vi "Lift Joystick Get.vi"(8 "Button Index's":T2, 9 "Setpoints":T1, 10 "Joystick IN":bool[](array[boolean]), 11 "Position IN":dbl format="%#_13g") -> (2 "Which Button?":i32, 3 "Position":dbl)   [LabVIEW 2014]
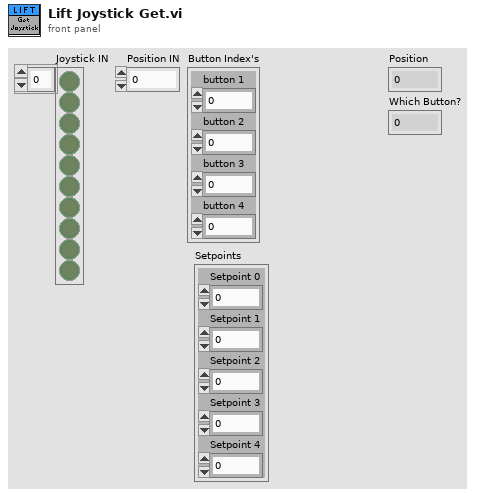
[diagram p1: front panel]
types:
  T1 = cluster{"Setpoint 0":dbl, "Setpoint 1":dbl, "Setpoint 2":dbl, "Setpoint 3":dbl, "Setpoint 4":dbl}
  T2 = cluster{"button 1":i32, "button 2":i32, "button 3":i32, "button 4":i32}
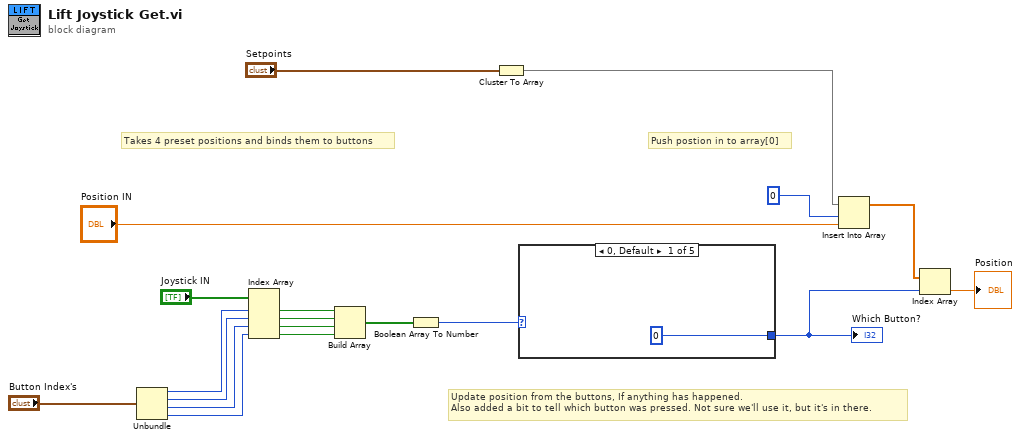
[diagram p0: block diagram]
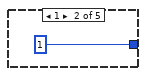
[diagram p2: hidden frame]
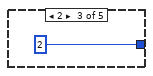
[diagram p3: hidden frame]
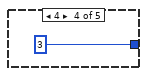
[diagram p4: hidden frame]
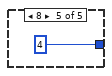
[diagram p5: hidden frame]
diagram:
  # "Push postion in to array[0]"
  # "Takes 4 preset positions and binds them to buttons"
  # "Update position from the buttons, If anything has happened.\nAlso added a bit to tell which button was pressed. Not sure we'll use it, but it's in there."
  n1 = Unbundle("Button Index's") -> ("button 1"=w17:i32, "button 2"=w16:i32, "button 3"=w15:i32, "button 4"=w14:i32)
  n2 = Index Array(array="Joystick IN", index #1=w17, index #2=w16, index #3=w15, index #4=w14) -> (element #1=w10:bool, element #2=w11:bool, element #3=w12:bool, element #4=w13:bool)
  n3 = Build Array(w10, w11, w12, w13) -> (w9:bool[])
  n4 = Boolean Array To Number(Boolean array=w9) -> (number=w8:u32)
  n5 = Cluster To Array(cluster="Setpoints") -> (array=w7:dbl[])
  n6 = case shown="0, Default" w8 {
    tunnel: [0 1 2 3 4] -> w4
    frame 0, Default {
    }
    frame 1 {
    }
    frame 2 {
    }
    frame 4 {
    }
    frame 8 {
    }
  }
  "Which Button?" <- w4
  n7 = Insert Into Array(array=w7, index=0, new element="Position IN") -> (w3:dbl[])
  n8 = Index Array(array=w3, index=w4) -> (element=→"Position":dbl)
